vi "Set Lamp.vi"(0 "comm interface in":refnum<class "Pixy Com.lvclass">, 5 "lamp enable":cluster{"upper":bool, "lower":bool}, 11 "error in":errorcluster) -> (4 "comm interface out":refnum<class "Pixy Com.lvclass">, 15 "error out":errorcluster)   [LabVIEW 2018, in "Pixy2.lvlib"]
uses:
  Pixy2.lvlib
  Interface/Pixy Com.lvclass
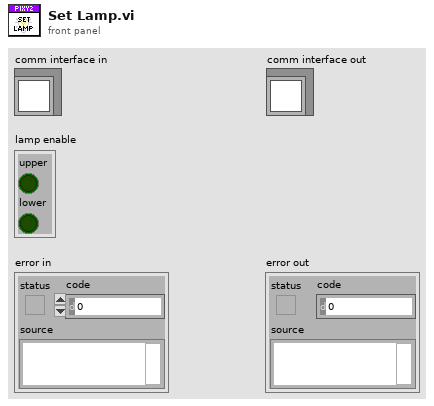
[diagram p1: front panel]
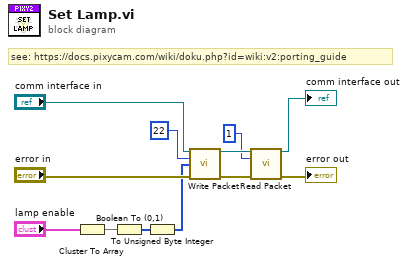
[diagram p0: block diagram]
diagram:
  # "see: https://docs.pixycam.com/wiki/doku.php?id=wiki:v2:porting_guide"
  n1 = Cluster To Array(cluster="lamp enable") -> (array=w4:bool[])
  n2 = Boolean To (0,1)(Boolean=w4) -> (0, 1=w3:i16[])
  n3 = To Unsigned Byte Integer(number=w3) -> (unsigned 8bit integer=w2:u8[])
  n4 = call "Write Packet.vi"("comm interface in"="comm interface in", "type"=u8 22, "payload"=w2, "error in"="error in") -> ("comm interface out"=w9:refnum<class "Pixy Com.lvclass">, "error out"=w10:errorcluster)  [unwired: 10 in]
  n5 = call "Read Packet.vi"("comm interface in"=w9, "expected type"=u8 1, "error in"=w10) -> ("comm interface out"=→"comm interface out":refnum<class "Pixy Com.lvclass">, "error out"=→"error out":errorcluster)  [unwired: 9 in, 2 out]
